vi "TL_experiment_path_definition.vi"(3 "error in":errorcluster, 4 "Path to the time lapse saving folder":path, 5 "data":cluster{"Channel":string, "ROI #":i32}) -> (0 "error out":errorcluster, 1 "time file path":path, 2 "movie path":path)   [LabVIEW 2015]
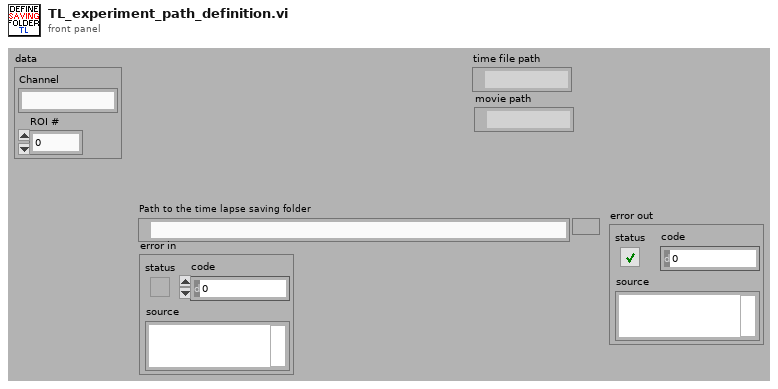
[diagram p1: front panel]
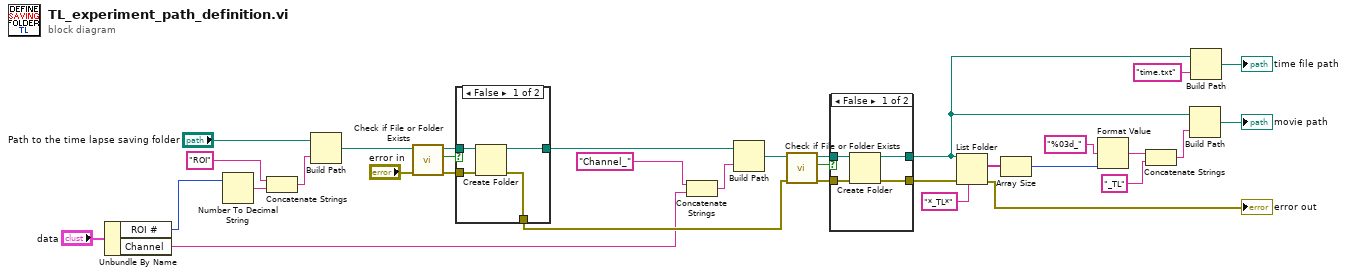
[diagram p0: block diagram]
diagram:
  n1 = Unbundle By Name("data") -> ("ROI #"=w11:i32, "Channel"=w10:string)
  n2 = Number To Decimal String(number=w11) -> (decimal integer string=w28:string)  [unwired: 1 in]
  n3 = Concatenate Strings("ROI" ("string"), w28) -> (w27:string)
  n4 = Build Path(base path="Path to the time lapse saving folder", name or relative path=w27) -> (appended path=w26:path)
  n5 = call <vilib>:"Check if File or Folder Exists.vi"("error in (no error)"="error in", "path"=w26) -> ("error out"=w30:errorcluster, "file or folder exists?"=w31:bool, "dup path"=w32:path)  [unwired: 7 in]
  n6 = case shown="False" w31 {
    tunnel: w30 -> [w37 w39]
    tunnel: w32 -> [w36 w38]
    tunnel: [w35 w39] -> w15
    tunnel: [w34 w38] -> w21
    frame False {
      n7 = Create Folder(path (use dialog)=w36, error in=w37) -> (created path=w34:path, error out=w35:errorcluster)  [unwired: 1 in, 1 out]
    }
    frame True {
    }
  }
  n8 = Concatenate Strings("Channel_" ("string"), w10) -> (w20:string)
  n9 = Build Path(base path=w21, name or relative path=w20) -> (appended path=w16:path)
  n10 = call <vilib>:"Check if File or Folder Exists.vi"("error in (no error)"=w15, "path"=w16) -> ("error out"=w19:errorcluster, "file or folder exists?"=w18:bool, "dup path"=w17:path)  [unwired: 7 in]
  n11 = case shown="False" w18 {
    tunnel: w19 -> [w43 w44]
    tunnel: w17 -> [w42 w45]
    tunnel: [w41 w45] -> w5
    tunnel: [w40 w44] -> w9
    frame False {
      n12 = Create Folder(path (use dialog)=w42, error in=w43) -> (created path=w41:path, error out=w40:errorcluster)  [unwired: 1 in, 1 out]
    }
    frame True {
    }
  }
  n13 = List Folder(path=w5, pattern="*_TL*", error in=w9) -> (filenames=w8:string[], error out=→"error out":errorcluster)  [unwired: 1 in, 2 out]
  n14 = Array Size(array=w8) -> (size(s)=w7:i32)
  n15 = Format Value(format string="%03d_", value (0)=w7) -> (output string=w24:string)  [unwired: 1 in]
  n16 = Concatenate Strings(w24, "_TL" ("string")) -> (w22:string)
  n17 = Build Path(base path=w5, name or relative path=w22) -> (appended path=→"movie path":path)
  n18 = Build Path(base path=w5, name or relative path="time.txt") -> (appended path=→"time file path":path)
